vi "Save Animated GIF Image (Memory).vi"(7 "Dither (None)":T2, 8 "error in (no error)":errorcluster, 9 "Delays":i32[](array[numeric]), 10 "Frames":T1[](array[typedef])) -> (0 "error out":errorcluster, 3 "Encoded Image":u8[](array[numeric]))   [LabVIEW 2020, in "G-Image.lvlib"]
doc: "Saves a sequences of images in animated GIF format to disk.\n\nTrue color images will be automatically quantized to 8-bit using a median-cut filter, and optional dithering. This process can be slow for large images."
uses:
  G-Image.lvlib
  <vilib>/picture/picture.llb/imagedata.ctl
  Controls/Dither Type.ctl
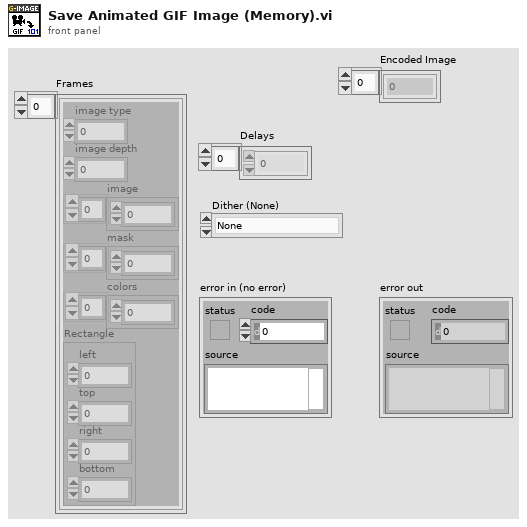
[diagram p1: front panel]
types:
  T1 = typedef "imagedata.ctl" = cluster{"image type":i32, "image depth":i32, "image":u8[], "mask":u8[], "colors":u32[], "Rectangle":cluster{"left":i16, "top":i16, "right":i16, "bottom":i16}}
  T2 = typedef "G-Image.lvlib/Dither Type.ctl" = enum32{"None", "Floyd-Steinberg"}
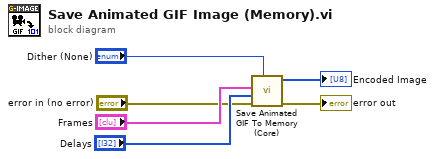
[diagram p0: block diagram]
diagram:
  n1 = call "Save Animated GIF To Memory (Core).vi"("Dither (None)"="Dither (None)", "error in (no error)"="error in (no error)", "Delays"="Delays", "Frames"="Frames") -> ("error out"=→"error out":errorcluster, "Encoded Image"=→"Encoded Image":u8[])  [unwired: 6 in]
